vi "Construct Connection Manager.vi"(5 "ID":string, 6 "ProtectedConnectionReader":refnum<class "ProtectedConnectionReader.lvclass">, 7 "Log Instance":refnum<class "LoggerReference.lvclass">, 8 "ProtectedConnectionWriter":refnum<class "ProtectedConnectionWriter.lvclass">, 9 "Message Return Policy":refnum<class "IMessageReturnPolicy.lvclass">, 10 "Write Policy":refnum<class "IWriteStrategy.lvclass">, 11 "Read Policy":refnum<class "IReadStrategy.lvclass">) -> (3 "ConnectionManager out":refnum<class "ConnectionManager.lvclass">)   [LabVIEW 2019, in "ConnectionManager.lvlib" / "ConnectionManager.lvclass"]
uses:
  <vilib>/gpm_packages/@cs/Network-interface/Source/ConnectionManager/ConnectionManager/ConnectionManager.lvclass
  C:/Program Files/National Instruments/LabVIEW 2019/vi.lib/gpm_packages/@cs/Network-interface/Source/Logged Actor/LoggedActor.lvclass
  <vilib>/gpm_packages/@cs/Network-interface/Source/MessagingInterfaces/IReadStrategy/IReadStrategy.lvclass
  <vilib>/gpm_packages/@cs/Network-interface/Source/MessagingInterfaces/IWriteStrategy/IWriteStrategy.lvclass
  <vilib>/gpm_packages/@cs/Network-interface/Source/MessagingInterfaces/IMessageReturnPolicy/IMessageReturnPolicy.lvclass
  <vilib>/gpm_packages/@cs/Network-interface/Source/ProtectedConnectionWriter/ProtectedConnectionWriter.lvclass
  <vilib>/gpm_packages/@cs/Network-interface/Source/ProtectedConnectionReader/ProtectedConnectionReader.lvclass
  <vilib>/gpm_packages/@cs/event-logger/Source/Composed Log/LoggerReference/LoggerReference.lvclass
  <vilib>/gpm_packages/@cs/Network-interface/Source/ConnectionManager/ConnectionManager/ConnectionManager.lvclass/ConnectionManager.ctl
  <vilib>/gpm_packages/@cs/Network-interface/Source/Logged Actor/LoggedActor.lvclass/LoggedActor.ctl
  <vilib>/gpm_packages/@cs/Network-interface/Source/Logged Actor/LoggedActor.lvclass
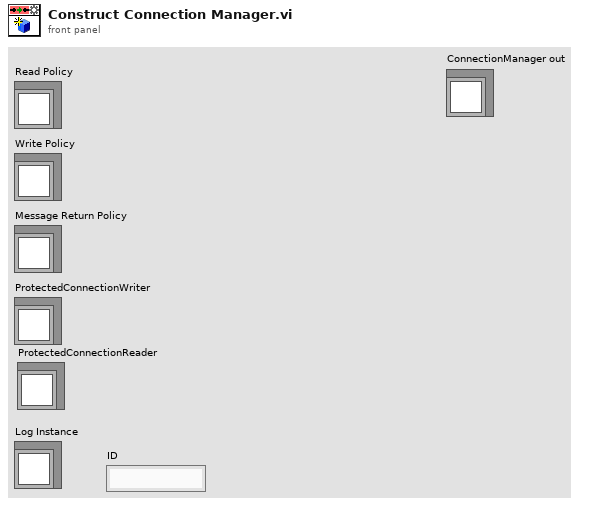
[diagram p1: front panel]
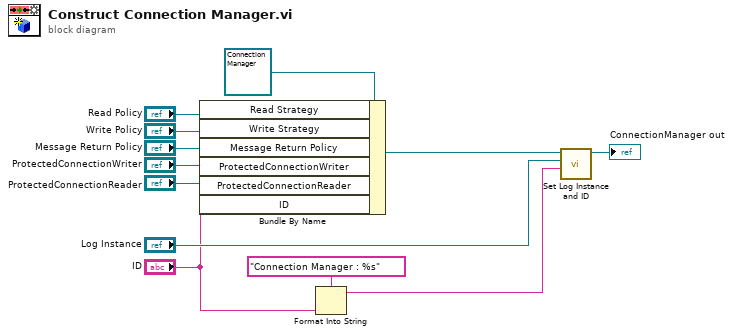
[diagram p0: block diagram]
diagram:
  n1 = Bundle By Name(cluster=refnum<class "ConnectionManager.lvclass"> refnum ("ConnectionManager in"), "Read Strategy"="Read Policy", "Write Strategy"="Write Policy", "Message Return Policy"="Message Return Policy", "ProtectedConnectionWriter"="ProtectedConnectionWriter", "ProtectedConnectionReader"="ProtectedConnectionReader", "ID"="ID") -> (w6:refnum<class "ConnectionManager.lvclass">)
  n2 = Format Into String(format string="Connection Manager : %s", "ID") -> (resulting string=w1:string)  [unwired: 2 in, 1 out]
  n3 = call <vilib>:"Set Log Instance and ID.vi"("Log Alias"=w1, "Log Instance"="Log Instance", "LoggedActor in"=w6) -> ("LoggedActor out"=→"ConnectionManager out":refnum<class "ConnectionManager.lvclass">)  [unwired: 8 in]
